vi "TCP Write to Connection.vi"(5 "Options":T1={"Ignore Timeout Error"=FALSE, "timeout ms (1000)"=1000}, 7 "error in":errorcluster, 8 "index":i32, 9 "Variant":variant, 10 "Meta data Name":string) -> (0 "error out":errorcluster)   [LabVIEW 2014, in "QwaveSys Raspberry Pi Library.lvlib"]
doc: "This VI writes a package of data to the connection specified by \"index\". It also prepends a specified meta data ID to each packet. \n\nThis VI is responsible for flattening the desired data to a string before transmission."
uses:
  QwaveSys Raspberry Pi Library.lvlib
  TCP/stm_TCP Write Options.ctl
  stm_TCPConnectionMethod.ctl
  TCP/STM Write Message (TCP).vi
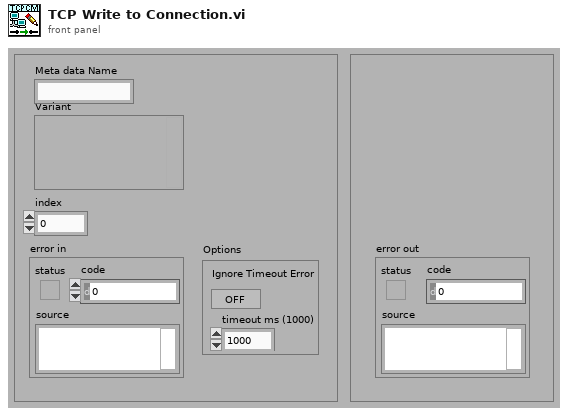
[diagram p1: front panel]
types:
  T1 = typedef "QwaveSys Raspberry Pi Library.lvlib/stm_TCP Write Options.ctl" = cluster{"Ignore Timeout Error":bool, "timeout ms (1000)":i32}
  T2 = typedef "QwaveSys Raspberry Pi Library.lvlib/stm_TCPConnectionMethod.ctl" = enum16{"Initialize", "Add Connection", "Set Properties", "Get Connection(s)", "Remove Connection", "Remove All Connections", "Get Connection Count"}
  T3 = typedef "QwaveSys Raspberry Pi Library.lvlib/stm_TCP Connection Info.ctl" = cluster{"connection ID":refnum<k5>, "Meta data":T4[]}
  T4 = typedef "QwaveSys Raspberry Pi Library.lvlib/stm_MetaDataElement.ctl" = string
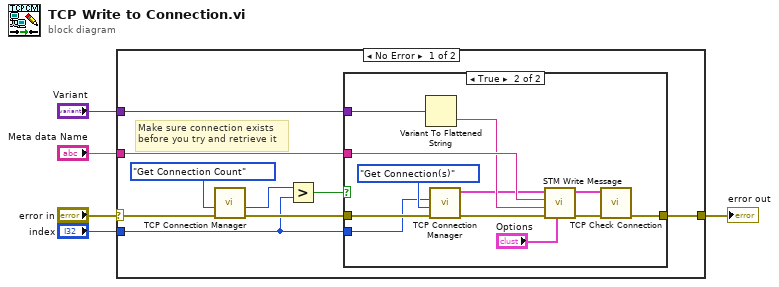
[diagram p0: block diagram]
diagram:
  n1 = case shown="No Error" "error in" {
    selector: "error in" -> [w9 w28]
    tunnel: "Variant" -> [w14 _]
    tunnel: "Meta data Name" -> [w13 _]
    tunnel: [w12 w28] -> w3
    tunnel: "index" -> [w6 _]
    frame No Error {
      # "Make sure connection exists\nbefore you try and retrieve it"
      n2 = call "TCP Connection Manager.vi"("error in (no error)"=w9, "Method"=stm_TCPConnectionMethod."Get Connection Count") -> ("error out"=w10:errorcluster, "Number of Connections"=w8:i32)  [unwired: 3 in, 5 out]
      n3 = Greater?(x=w8, y=w6) -> (0:w7:bool)
      n4 = case shown="True" w7 {
        tunnel: w10 -> [w15 w18]
        tunnel: [w15 w27] -> w12
        tunnel: w13 -> [_ w25]
        tunnel: w14 -> [_ w24]
        tunnel: w6 -> [_ w16]
        frame False {
        }
        frame True {
          n5 = Variant To Flattened String(Variant=w24) -> (data string=w23:string)  [unwired: 1 out]
          n6 = call "TCP Connection Manager.vi"("error in (no error)"=w18, "Method"=stm_TCPConnectionMethod."Get Connection(s)", "Index"=w16) -> ("error out"=w17:errorcluster, "Connection Out"=w19:T3)  [unwired: 2 in, 5 out]
          n7 = call-poly "STM Write Message.vi"("Options"="Options", "error in (no error)"=w17, "Data"=w23, "Name"=w25, "Connection Info"=w19) -> ("error out"=w22:errorcluster, "Connection Info Out"=w26:T3)  [unwired: 5 out]
          n8 = call "TCP Check Connection.vi"("error in (no error)"=w22, "Connection In"=w26) -> ("error out"=w27:errorcluster)  [unwired: 9 out]
        }
      }
    }
    frame Error {
    }
  }
  "error out" <- w3
